vi "GenerateFileName.vi"(4 "error in (no error)":errorcluster, 6 "FileExtension":string, 7 "SampleName":string) -> (0 "error out":errorcluster, 2 "FilePathOut":path, 3 "FolderNameString":string)   [LabVIEW 2014]
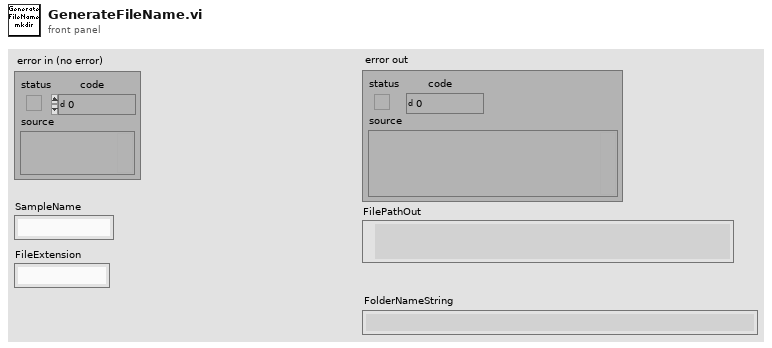
[diagram p1: front panel]
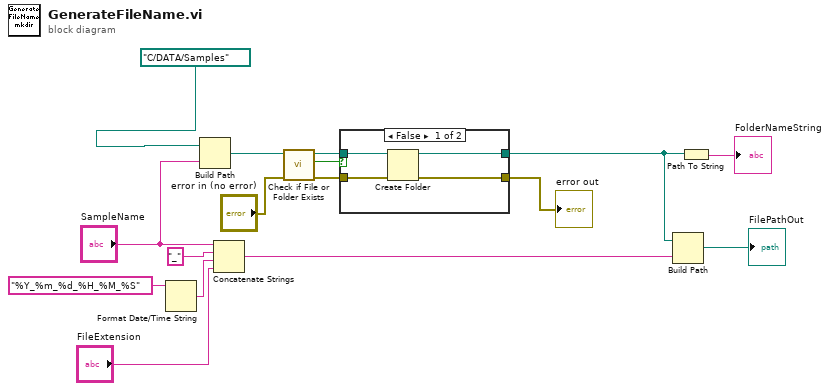
[diagram p0: block diagram]
diagram:
  n1 = Format Date/Time String(time format string (%c)="%Y_%m_%d_%H_%M_%S") -> (date/time string=w14:string)  [unwired: 2 in]
  n2 = Build Path(base path=path "C:/DATA/Samples" ("Path"), name or relative path="SampleName") -> (appended path=w8:path)
  n3 = Concatenate Strings("SampleName", "_", w14, "FileExtension") -> (w11:string)
  n4 = call <vilib>:"Check if File or Folder Exists.vi"("error in (no error)"="error in (no error)", "path"=w8) -> ("error out"=w6:errorcluster, "file or folder exists?"=w9:bool, "dup path"=w7:path)  [unwired: 7 in]
  n5 = case shown="False" w9 {
    tunnel: w7 -> [w20 w22]
    tunnel: [w19 w22] -> w3
    tunnel: w6 -> [w18 w21]
    tunnel: [w17 w21] -> w4
    frame False {
      n6 = Create Folder(path (use dialog)=w20, error in=w18) -> (created path=w19:path, error out=w17:errorcluster)  [unwired: 1 in, 1 out]
    }
    frame True {
    }
  }
  "error out" <- w4
  n7 = Build Path(base path=w3, name or relative path=w11) -> (appended path=→"FilePathOut":path)
  n8 = Path To String(path=w3) -> (string=→"FolderNameString":string)
